vi "disk_getRelativePath.vi"(8 "error in (no error)":errorcluster, 9 "temp folder":path, 10 "absolute path":path) -> (0 "error out":errorcluster, 1 "relative path out":path, 2 "absolute path out":path)   [LabVIEW 2020, in "NI_ExcelFile.lvlib"]
uses:
  <vilib>/express/express shared/NI_ExcelFile/NI_ExcelFile.lvlib
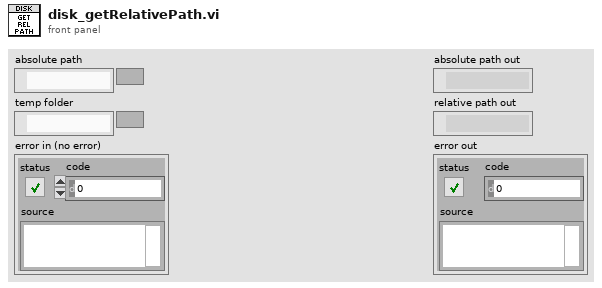
[diagram p1: front panel]
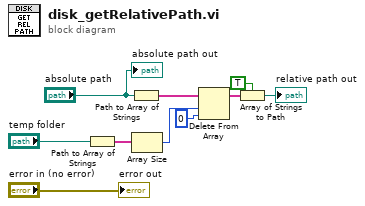
[diagram p0: block diagram]
diagram:
  n1 = Path to Array of Strings(0:"temp folder") -> (2:w7:string[])  [unwired: 1 out]
  n2 = Path to Array of Strings(0:"absolute path") -> (2:w10:string[])  [unwired: 1 out]
  n3 = Array Size(array=w7) -> (size(s)=w6:i32)
  n4 = Delete From Array(array=w10, length=w6, index=0) -> (array with subset deleted=w4:string[])  [unwired: 1 out]
  n5 = Array of Strings to Path(0:w4, 1:TRUE ("relative")) -> (2:→"relative path out":path)
  "absolute path out" <- "absolute path"
  "error out" <- "error in (no error)"
